vi "take snapshot.vi"(8 "error in (no error)":errorcluster, 10 "take snapshot":bool, 11 "vi ref":refnum<vi>) -> (0 "error out":errorcluster)   [LabVIEW 2017]
uses:
  popup panels/control panel globals.vi
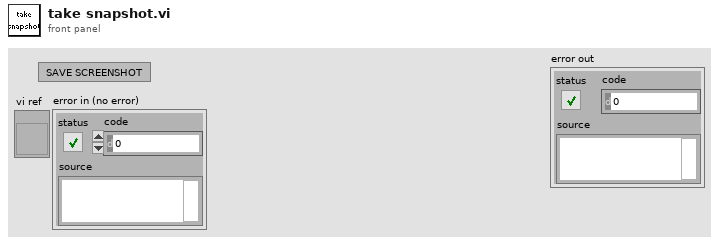
[diagram p1: front panel]
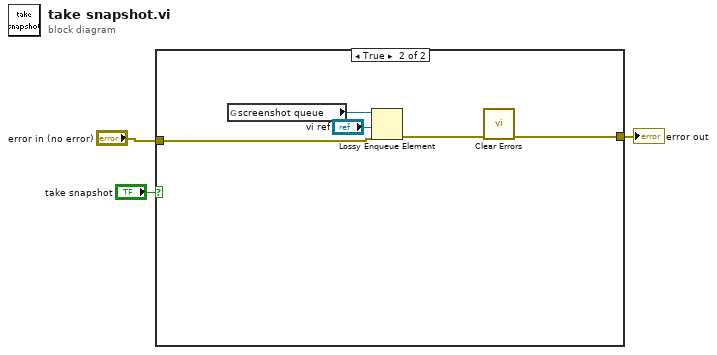
[diagram p0: block diagram]
diagram:
  n1 = case shown="True" "take snapshot" {
    tunnel: "error in (no error)" -> [w4 w7]
    tunnel: [w4 w5] -> w1
    frame False {
    }
    frame True {
      n2 = global read "control panel globals.vi" "screenshot queue"() -> (w9:refnum<queue>)
      n3 = Lossy Enqueue Element(queue=w9, element="vi ref", error in (no error)=w7) -> (error out=w6:errorcluster)  [unwired: 3 out]
      n4 = call <vilib>:"Clear Errors.vi"("error in (no error)"=w6) -> ("error out"=w5:errorcluster)  [unwired: 5 in, 1 out]
    }
  }
  "error out" <- w1
